vi "testLocateNIDAQ.vi"() -> ()   [LabVIEW 2017]
uses:
  <resource>/objmgr/daqmx.rc
panel:
  out "AI.PhysicalChans":tag[](array[tag])
  out "Module":tag
  out "DevNamesIn":tag[](array[tag])
  out "DevNamesOut":tag[](array[tag])
  in  "Multicolumn Listbox":i32(listbox)
  out "error out":errorcluster
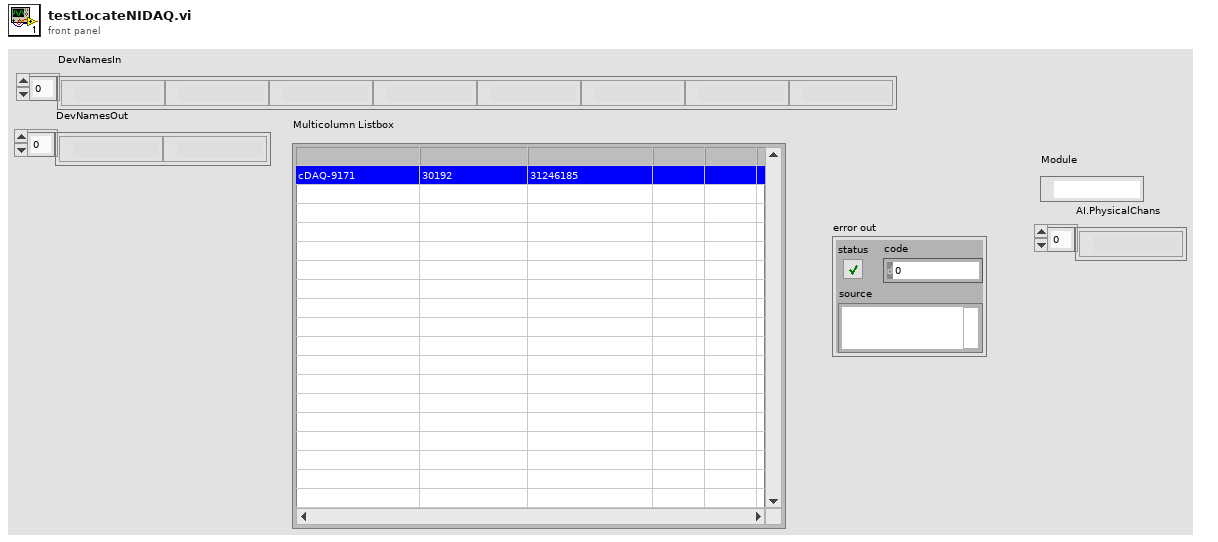
[diagram p1: front panel]
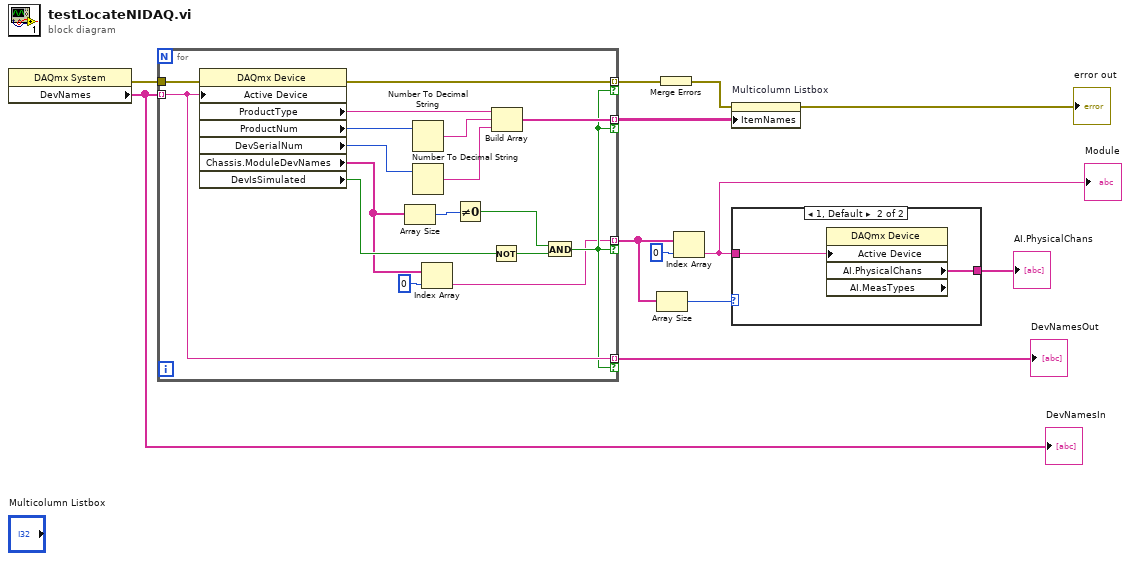
[diagram p0: block diagram]
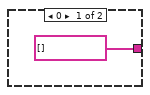
[diagram p2: hidden frame]
diagram:
  n1 = property class="DAQmx System"() -> (error out=w10:errorcluster, "DevNames"=w12:tag[])  [unwired: 2 in, 1 out]
  "DevNamesIn" <- w12
  n2 = for {
    tunnel: w12 -> [w17] mode=indexing
    tunnel: [w27] -> w11 mode=indexing if=w14
    tunnel: [w13] -> w3 mode=indexing if=w14
    tunnel: w10 -> [w23]
    tunnel: [w22] -> w8 mode=indexing if=w14
    tunnel: [w17] -> w6 mode=indexing if=w14
    n3 = property class="DAQmx Device"(error in=w23, "Active Device"=w17) -> (error out=w22:errorcluster, "ProductType"=w28:string, "ProductNum"=w29:u32, "DevSerialNum"=w25:u32, "Chassis.ModuleDevNames"=w16:tag[], "DevIsSimulated"=w21:bool)  [unwired: 1 in, 1 out]
    n4 = Array Size(array=w16) -> (size(s)=w20:i32)
    n5 = Number To Decimal String(number=w29) -> (decimal integer string=w26:string)  [unwired: 1 in]
    n6 = Number To Decimal String(number=w25) -> (decimal integer string=w24:string)  [unwired: 1 in]
    n7 = Index Array(array=w16, index=0) -> (element=w13:tag)
    n8 = Not Equal To 0?(x=w20) -> (x != 0?=w19:bool)
    n9 = Not(x=w21) -> (.not. x?=w18:bool)
    n10 = Build Array(w28, w26, w24) -> (w27:string[])
    n11 = And(x=w19, y=w18) -> (x .and. y?=w14:bool)
  }
  "DevNamesOut" <- w6
  n12 = Array Size(array=w3) -> (size(s)=w5:i32)
  n13 = Merge Errors(w8) -> (w7:errorcluster)
  n14 = Index Array(array=w3, index=0) -> (element=w1:tag)
  "Module" <- w1
  n15 = property on="Multicolumn Listbox" class="MCListbox (strict)"(error in=w7, "ItemNames"=w11) -> (error out=→"error out":errorcluster)  [unwired: 1 in, 1 out]
  n16 = case shown="1, Default" w5 {
    tunnel: [tag[] [] ("AI.PhysicalChans") w32] -> w4
    tunnel: w1 -> [_ w31]
    frame 0 {
    }
    frame 1, Default {
      n17 = property class="DAQmx Device" props=["Active Device", "AI.PhysicalChans", "AI.MeasTypes"]("Active Device"=w31) -> ("AI.PhysicalChans"=w32:tag[])  [unwired: 2 in, 3 out]
    }
  }
  "AI.PhysicalChans" <- w4
